vi "RogersLog.vi"(0 "Text to add":string, 1 "ROS":T3={"topic port"=0, "Node"="", "topic"="", "type"="", "node port"=0, "error "={"status"=FALSE, "code"=0, "source"=""}, "Direction"=enum."Node", "Update (ms)"=1, "FIFO size"=0}, 2 "Log":T2={"Sent"="", "Reply"="", "MethodName"="", "success"=TRUE, "Dir1"="", "Dir2"="", "Time Stamp"="", "error"={"status"=FALSE, "code"=0, "source"=""}, "Preamble"="", "Midamble"="", "Postamble"=""}, 3 "LogPath in":path, 4 "Task":T1(ring)=enum."Add Task") -> (5 "HTML":string, 6 "LogPath out":path)   [LabVIEW 2015]
uses:
  _ROSControl.ctl
  _ROSDirection.ctl
  Console/Servers/ServerSubs/ROSLog.ctl
  _ROSDefinition.vi
panel:
  out "Counter":i32
  # "First line is the Menu name - rest is a reamble."
  # "Changed log typedef and then all the registrations"
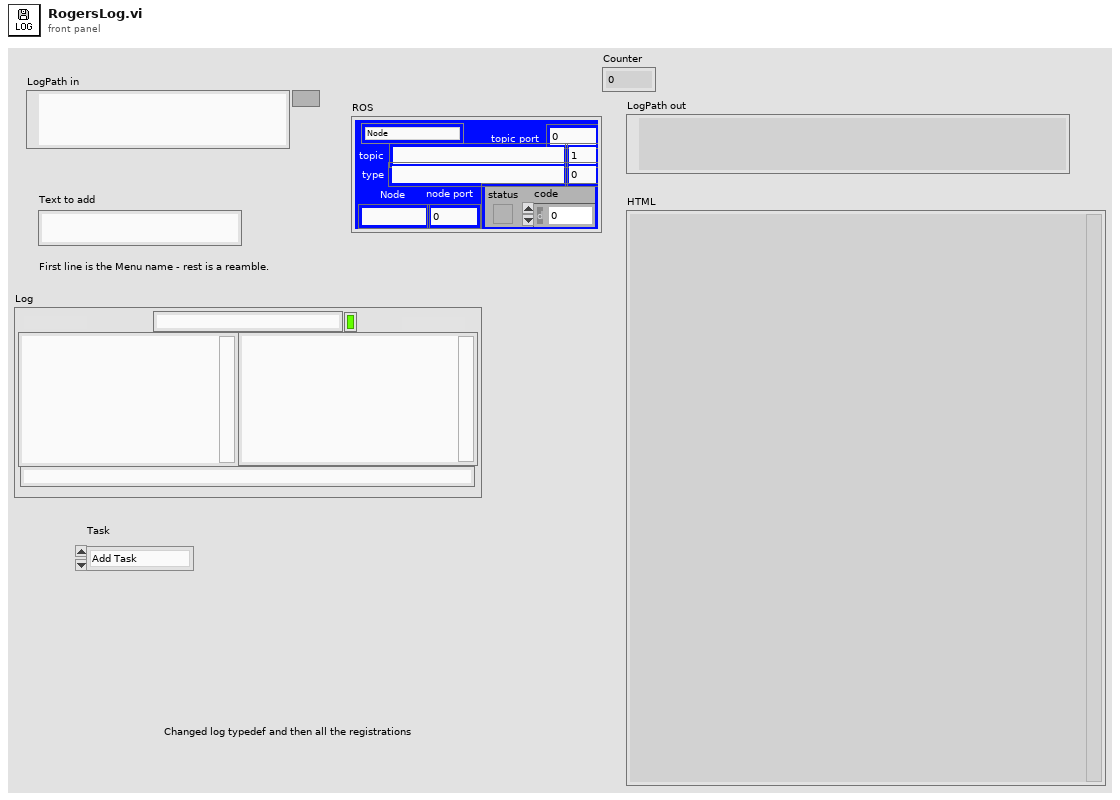
[diagram p1: front panel]
types:
  T1 = enum16{"Reset Log", "Add Client", "Remove Client", "Add Task"}
  T2 = typedef "ROSLog.ctl" = cluster{"Sent":string, "Reply":string, "MethodName":string, "success":bool, "Dir1":string, "Dir2":string, "Time Stamp":string, "error":errorcluster, "Preamble":string, "Midamble":string, "Postamble":string}
  T3 = typedef "_ROSControl.ctl" = cluster{"topic port":u16, "Node":string, "topic":string, "type":string, "node port":u16, "error ":errorcluster, "Direction":T4, "Update (ms)":u16, "FIFO size":u16}
  T4 = typedef "_ROSDirection.ctl" = enum16{"Node", "Publisher", "Subscriber", "ServiceClient", "ServiceProvider"}
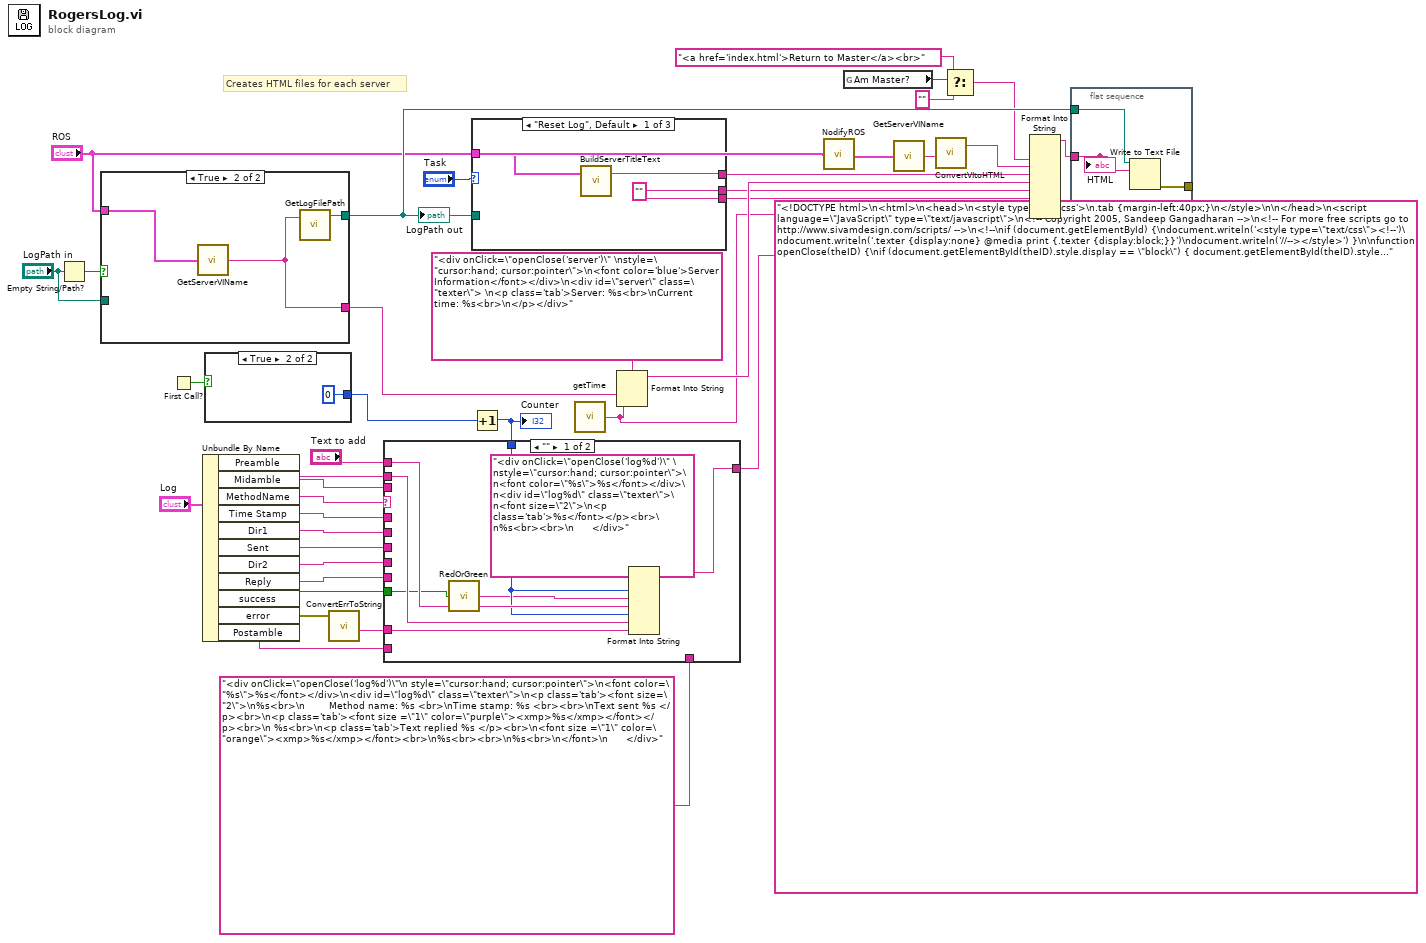
[diagram p0: block diagram]
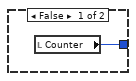
[diagram p2: hidden frame]
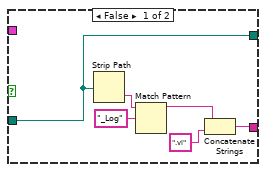
[diagram p3: hidden frame]
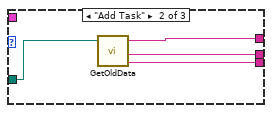
[diagram p4: hidden frame]
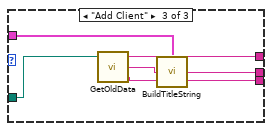
[diagram p5: hidden frame]
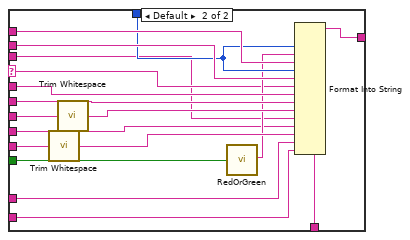
[diagram p6: hidden frame]
diagram:
  # "Creates HTML files for each server"
  n1 = Empty String/Path?(string/path="LogPath in") -> (empty?=w24:bool)
  n2 = case shown="True" w24 {
    tunnel: [w43 w47] -> w19
    tunnel: "LogPath in" -> [w46 _]
    tunnel: [w46 w49] -> w22
    tunnel: "ROS" -> [_ w48]
    frame False {
      n3 = Strip Path(path=w46) -> (name=w45:string)  [unwired: 1 out]
      n4 = Match Pattern(string=w45, regular expression="_Log") -> (before substring=w42:string)  [unwired: 1 in, 3 out]
      n5 = Concatenate Strings(w42, ".vi" ("regular expression")) -> (w43:string)
    }
    frame True {
      n6 = call "GetServerVIName.vi"("ROS"=w48) -> ("vi name"=w47:string)
      n7 = call "GetLogFilePath.vi"("Server name"=w47) -> ("LogPath"=w49:path)  [unwired: 1 in, 1 out]
    }
  }
  "LogPath out" <- w22
  n8 = First Call?() -> (First Call?: T/F=w17:bool)
  n9 = Unbundle By Name("Log") -> ("Preamble"=w13:string, "Midamble"=w12:string, "MethodName"=w20:string, "Time Stamp"=w37:string, "Dir1"=w36:string, "Sent"=w35:string, "Dir2"=w34:string, "Reply"=w33:string, "success"=w28:bool, "error"=w15:errorcluster, "Postamble"=w11:string)
  n10 = case shown="True" w17 {
    tunnel: [w50 0 ("Counter")] -> w16
    frame False {
      n11 = local read "Counter"() -> (w50:i32)
    }
    frame True {
    }
  }
  n12 = call "ConvertErrToString.vi"("error in (no error)"=w15) -> ("String"=w14:string)  [unwired: 1 out]
  n13 = case shown="\"Reset Log\", Default" "Task" {
    tunnel: [w54 w55 w59] -> w29
    tunnel: [w53 w58 w64] -> w27
    tunnel: [w54 w56 w62] -> w25
    tunnel: w22 -> [_ w57 w63]
    tunnel: "ROS" -> [w52 _ w61]
    frame "Reset Log", Default {
      w54 = "" ("tagged text")
      n14 = call "BuildServerTitleText.vi"("ROS"=w52) -> ("colored text"=w53:string)  [unwired: 1 in, 1 out]
    }
    frame "Add Task" {
      n15 = call "GetOldData.vi"("LogPath"=w57) -> ("log"=w55:string, "clients"=w56:string, "server"=w58:string)  [unwired: 2 in]
    }
    frame "Add Client" {
      n16 = call "GetOldData.vi"("LogPath"=w63) -> ("log"=w59:string, "clients"=w60:string, "server"=w64:string)  [unwired: 2 in]
      n17 = call "BuildTitleString.vi"("tagged text"=w60, "ROS"=w61) -> ("String"=w62:string)
    }
  }
  n18 = Increment(x=w16) -> (x+1=w18:i32)
  "Counter" <- w18
  n19 = case shown="\"\"" w20 {
    selector: w20 -> [_ w75]
    tunnel: "<div onClick=\"openClose('log%d')\"\n style=\"cursor:hand; cursor:pointer\">\n<font color=\"%s\">%s</font></div>\n<div id=\"log%d\" class=\"texter\">\n<p class='tab'><font size=\"2\">\n%s<br>\n        Method name: %s <br>\nTime stamp: %s <br><br>\nText sent %s </p><br>\n<p class='tab'><font size =\"1\" color=\"purple\"><xmp>%s</xmp></font></p><br>\n %s<br>\n<p class='tab'>Text replied %s </p><br>\n<font size =\"1\" color=\"orange\"><xmp>%s</xmp></font><br>\n%s<br><br>\n%s<br>\n</font>\n      </div>" ("regular expression") -> [_ w90]
    tunnel: w37 -> [_ w89]
    tunnel: w36 -> [_ w88]
    tunnel: w35 -> [_ w87]
    tunnel: w34 -> [_ w76]
    tunnel: w33 -> [_ w86]
    tunnel: [w72 w85] -> w2
    tunnel: w28 -> [w67 w84]
    tunnel: "Text to add" -> [w70 w83]
    tunnel: w13 -> [w69 w80]
    tunnel: w18 -> [w66 w79]
    tunnel: w14 -> [w68 w77]
    tunnel: w12 -> [_ w74]
    tunnel: w11 -> [_ w73]
    frame "" {
      n20 = call "RedOrGreen.vi"("success"=w67) -> ("color"=w65:string)
      n21 = Format Into String(format string="<div onClick=\"openClose('log%d')\" \nstyle=\"cursor:hand; cursor:pointer\">\n<font color=\"%s\">%s</font></div>\n<div id=\"log%d\" class=\"texter\">\n<font size=\"2\">\n<p class='tab'>%s</font></p><br>\n%s<br><br>\n      </div>" ("regular expression"), w66, w65, w70, w66, w69, w68) -> (resulting string=w72:string)  [unwired: 2 in, 1 out]
    }
    frame Default {
      n22 = call "Trim Whitespace.vi"("string"=w86) -> ("trimmed string"=w81:string)  [unwired: 1 in]
      n23 = call "Trim Whitespace.vi"("string"=w87) -> ("trimmed string"=w82:string)  [unwired: 1 in]
      n24 = call "RedOrGreen.vi"("success"=w84) -> ("color"=w78:string)
      n25 = Format Into String(format string=w90, w79, w78, w83, w79, w80, w75, w89, w88, w82, w74, w76, w81, w77, w73) -> (resulting string=w85:string)  [unwired: 2 in, 1 out]
    }
  }
  n26 = call "getTime.vi"() -> ("Current Time"=w1:string)  [unwired: 1 in]
  n27 = Format Into String(format string="<div onClick=\"openClose('server')\" \nstyle=\"cursor:hand; cursor:pointer\">\n<font color='blue'>Server Information</font></div>\n<div id=\"server\" class=\"texter\"> \n<p class='tab'>Server: %s<br>\nCurrent time: %s<br>\n</p></div>" ("regular expression"), w19, w1) -> (resulting string=w30:string)  [unwired: 2 in, 1 out]
  n28 = call "NodifyROS.vi"("ROS in"="ROS") -> ("ROS out"=w7:T3)
  n29 = global read "_ROSDefinition.vi" "Am Master?"() -> (w6:bool)
  n30 = call "GetServerVIName.vi"("ROS"=w7) -> ("vi name"=w10:string)
  n31 = call "ConvertVItoHTML.vi"("vi name"=w10) -> ("Htm log name"=w9:string)  [unwired: 1 out]
  n32 = Select(t="<a href='index.html'>Return to Master</a><br>" ("regular expression"), s=w6, f="") -> (s? t:f=w3:string)
  n33 = Format Into String(format string="<!DOCTYPE html>\n<html>\n<head>\n<style type='text/css'>\n.tab {margin-left:40px;}\n</style>\n\n</head>\n<script language=\"JavaScript\" type=\"text/javascript\">\n<!-- Copyright 2005, Sandeep Gangadharan -->\n<!-- For more free scripts go to http://www.sivamdesign.com/scripts/ -->\n<!--\nif (document.getElementById) {\ndocument.writeln('<style type=\"text/css\"><!--')\ndocument.writeln('.texter {display:none} @media print {.texter {display:block;}}')\ndocument.writeln('//--></style>') }\n\nfunction openClose(theID) {\nif (document.getElementById(theID).style.display == \"block\") { document.getElementById(theID).style.display = \"none\" }\nelse { document.getElementById(theID).style.display = \"block\" } }\n// -->\n</script>\n\n<body>\n%s\n<a href='%s'>Return to Node</a>\n<!----- start server ----->\n%s \n<!----- end server ----->\n \n%s\n<!----- start clients ----->\n%s\n<!----- end clients ----->\n<hr>\n<!----- start log ----->      \n%s\n%s (<font size=1>%s</font>)\n<!----- end log ----->\n\n<hr> For more help, go to the \n<a href=\"https://decibel.ni.com/content/groups/ros-for-labview?view=overview\">NI ROS community page</a> or \n<a href=\"https://github.com/tuftsBaxter/ROS-for-LabVIEW-Software\">the LVROS Github</a>\n\n</body>\n</html>" ("regular expression"), w3, w9, w27, w30, w25, w29, w2, w1) -> (resulting string=w31:string)  [unwired: 2 in, 1 out]
  n34 = flat-sequence {
    tunnel: w31 -> [w93]
    tunnel: w22 -> [w92]
    tunnel: [w91] -> _
    frame #0 {
      n35 = Write to Text File(file (use dialog)=w92, text=w93) -> (error out=w91:errorcluster)  [unwired: 2 in, 2 out]
      "HTML" <- w93
    }
  }
